vi "Add Named Gate Prefix.vi"(1 "name in":string) -> (0 "name out":string)   [LabVIEW 2015, in "Gates.lvlib"]
doc: "Adds \"CustomSemaphore.Gate.\" to the <b>name in</b>."
uses:
  Gates.lvlib
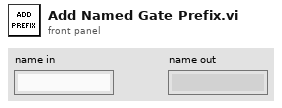
[diagram p1: front panel]
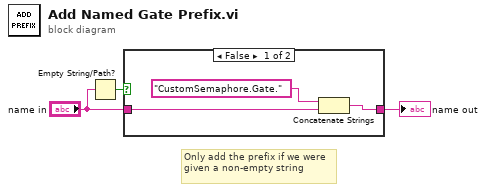
[diagram p0: block diagram]
diagram:
  # "Only add the prefix if we were given a non-empty string"
  n1 = Empty String/Path?(string/path="name in") -> (empty?=w3:bool)
  n2 = case shown="False" w3 {
    tunnel: "name in" -> [w6 w7]
    tunnel: [w4 w7] -> w1
    frame False {
      n3 = Concatenate Strings("CustomSemaphore.Gate." ("string"), w6) -> (w4:string)
    }
    frame True {
    }
  }
  "name out" <- w1
